vi "EnableCell.vi"(0 "Column in":refnum<class "Column.lvclass">, 5 "Cell Position":T1, 7 "Table Data in":string[][](array[string]), 9 "Table CtlRef In":refnum<vi>, 11 "error in (no error)":errorcluster) -> (4 "Column out":refnum<class "Column.lvclass">, 8 "Table Data out":string[][](array[string]), 10 "Table CtlRef Out":refnum<vi>, 15 "error out":errorcluster)   [LabVIEW 2013, in "Column.lvclass"]
uses:
  Column.lvclass
  <vilib>/Utility/miscctls.llb/LVRowAndColumnTypeDef.ctl
  Column.lvclass/Column.ctl
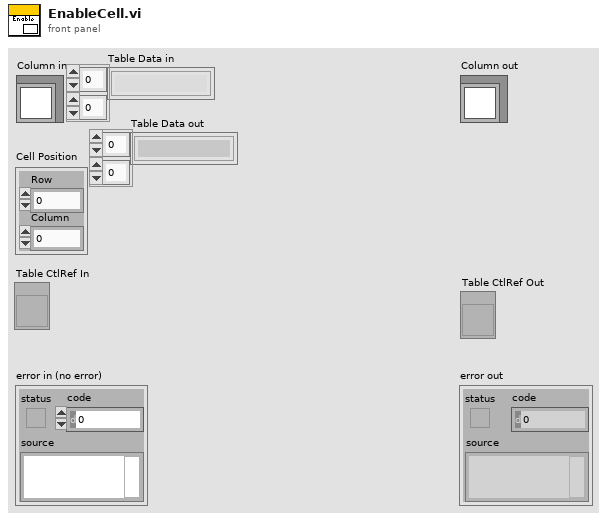
[diagram p1: front panel]
types:
  T1 = typedef "LVRowAndColumnTypeDef.ctl" = cluster{"Row":i32, "Column":i32}
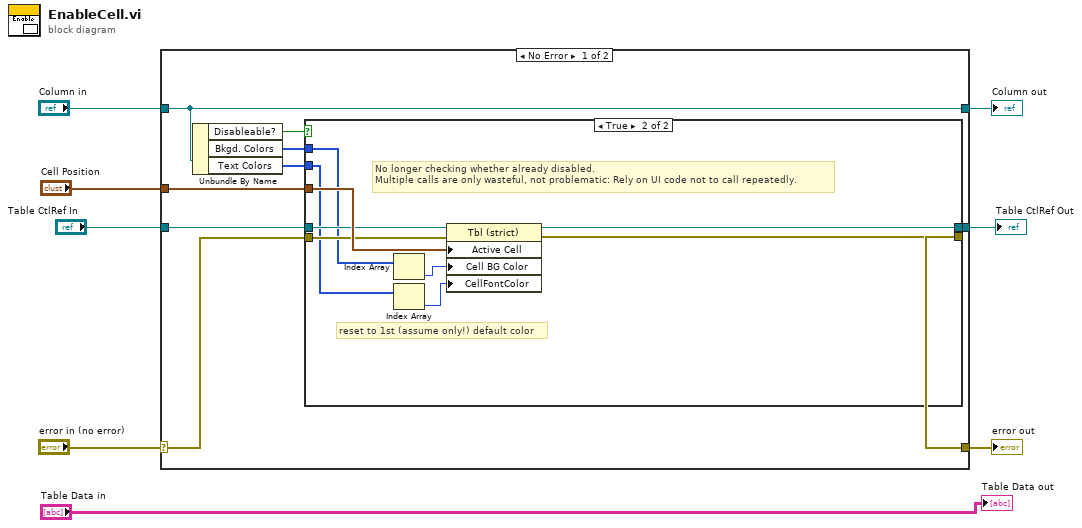
[diagram p0: block diagram]
diagram:
  n1 = case shown="No Error" "error in (no error)" {
    selector: "error in (no error)" -> [w14 w31]
    tunnel: [w13 w31] -> w7
    tunnel: [w12 w30] -> w5
    tunnel: "Column in" -> [w12 w30]
    tunnel: "Cell Position" -> [w15 _]
    tunnel: "Table CtlRef In" -> [w17 w29]
    tunnel: [w16 w29] -> w2
    frame No Error {
      n2 = Unbundle By Name(w12) -> ("Disableable?"=w11:bool, "Bkgd. Colors"=w10:u32[], "Text Colors"=w9:u32[])
      n3 = case shown="True" w11 {
        tunnel: w17 -> [w19 w25]
        tunnel: [w19 w28] -> w16
        tunnel: w15 -> [_ w27]
        tunnel: w14 -> [w18 w24]
        tunnel: [w18 w26] -> w13
        tunnel: w10 -> [_ w22]
        tunnel: w9 -> [_ w21]
        frame False {
          # "Do nothing if column must always be enabled!"
        }
        frame True {
          # "reset to 1st (assume only!) default color"
          # "No longer checking whether already disabled. \nMultiple calls are only wasteful, not problematic: Rely on UI code not to call repeatedly."
          n4 = Index Array(array=w22) -> (element=w23:u32)  [unwired: 1 in]
          n5 = Index Array(array=w21) -> (element=w20:u32)  [unwired: 1 in]
          n6 = property class="Tbl (strict)"(reference=w25, error in=w24, "Active Cell"=w27, "Cell BG Color"=w23, "CellFontColor"=w20) -> (reference out=w28:refnum<vi>, error out=w26:errorcluster)
        }
      }
    }
    frame Error {
    }
  }
  "error out" <- w7
  "Column out" <- w5
  "Table CtlRef Out" <- w2
  "Table Data out" <- "Table Data in"
